vi "Archive Errors.vi"(8 "Error In":errorcluster) -> (0 "error out":errorcluster)   [LabVIEW 2019]
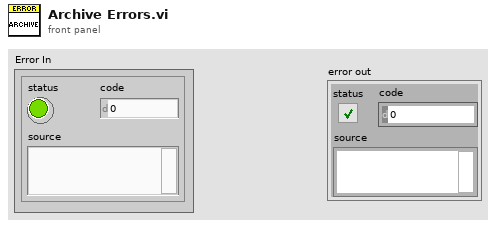
[diagram p1: front panel]
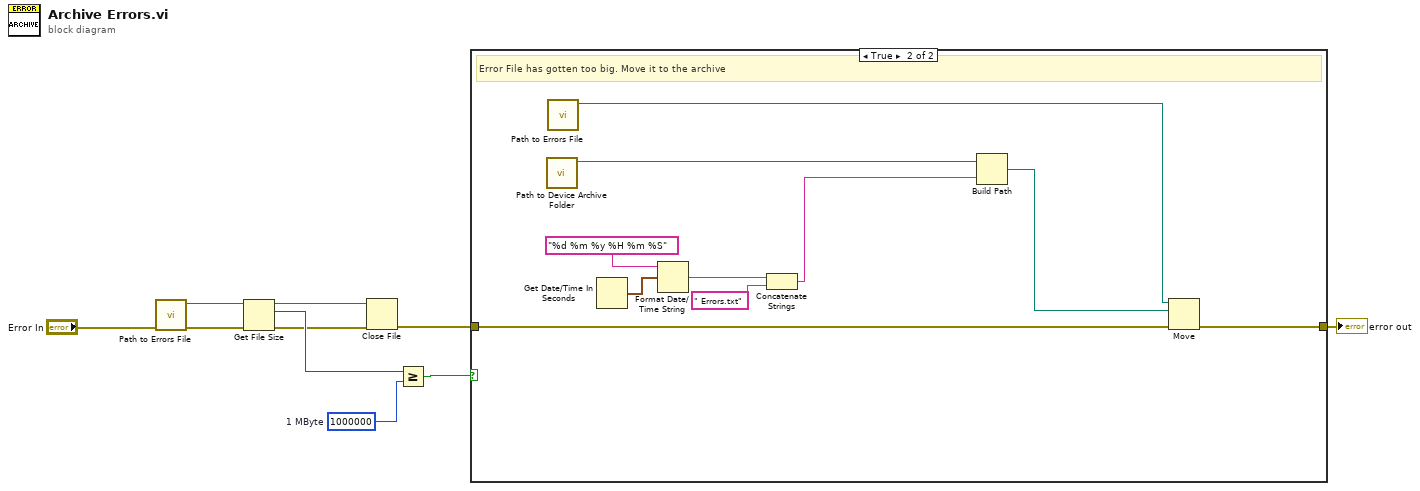
[diagram p0: block diagram]
diagram:
  w6 = i64 1000000  # 1 MByte
  n1 = call "Path to Errors File.vi"("Error In"="Error In") -> ("Error Out"=w8:errorcluster, "Path to Errors File"=w9:path)  [unwired: 9 in]
  n2 = Get File Size(file=w9, error in=w8) -> (refnum out=w4:refnum<file>, size (in bytes)=w7:i64, 0:w3:errorcluster)
  n3 = Close File(refnum=w4, error in=w3) -> (error out=w2:errorcluster)  [unwired: 1 out]
  n4 = Greater Or Equal?(x=w7, y=w6) -> (x >= y?=w5:bool)
  n5 = case shown="True" w5 {
    tunnel: w2 -> [w11 w20]
    tunnel: [w11 w12] -> w1
    frame False {
      # "Error file is still small so all good"
    }
    frame True {
      # "Error File has gotten too big. Move it to the archive"
      n6 = call "Path to Device Archive Folder.vi"() -> ("Path to Errors File"=w19:path)  [unwired: 10 in, 1 out]
      n7 = call "Path to Errors File.vi"() -> ("Path to Errors File"=w21:path)  [unwired: 10 in, 1 out]
      n8 = Get Date/Time In Seconds() -> (seconds since 1Jan1904=w18:timestamp)
      n9 = Format Date/Time String(time format string (%c)="%d %m %y %H %m %S", seconds (now)=w18) -> (date/time string=w16:string)  [unwired: 1 in]
      n10 = Concatenate Strings(w16, " Errors.txt" ("string")) -> (w14:string)
      n11 = Build Path(base path=w19, name or relative path=w14) -> (appended path=w13:path)
      n12 = Move(source path=w21, error in=w20, 10:w13) -> (error out=w12:errorcluster)  [unwired: 2 in, 2 out]
    }
  }
  "error out" <- w1
